vi "FMDLWaitKeithley6514ReadingBufferFull.vi"(0 "VISA resource name":refnum<visa-resource-name>, 1 "Timeout (10000 ms)":u32=10000, 2 "Buffer size previously set":i32, 3 "error in (no error)":errorcluster) -> (4 "Number of times the loop ran":i32, 5 "VISA resource name out":refnum<visa-resource-name>, 6 "Number of Readings in Buffer":i32, 7 "error out":errorcluster)   [LabVIEW 2018]
uses:
  <instrlib>/Keithley 6517/Keithley 6517.lvlib
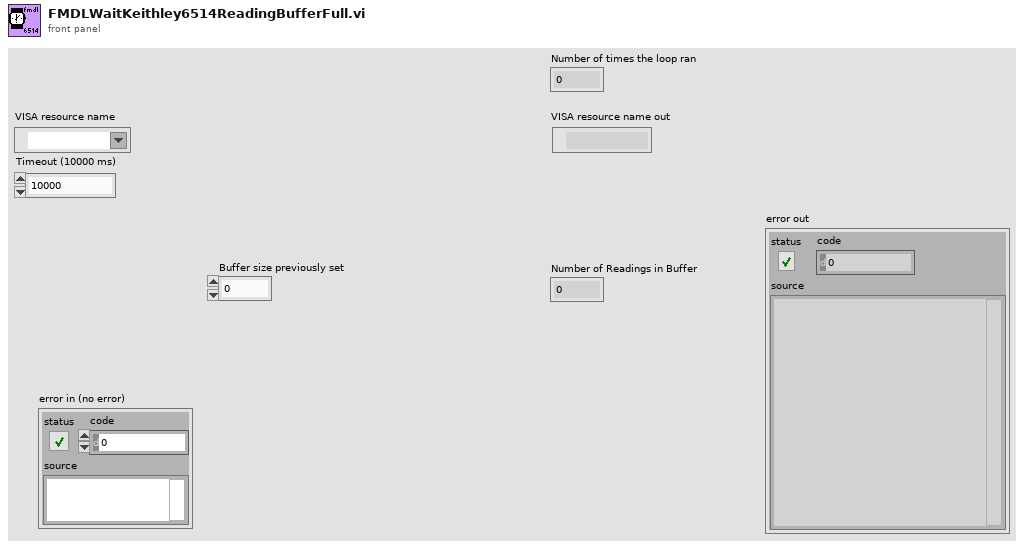
[diagram p1: front panel]
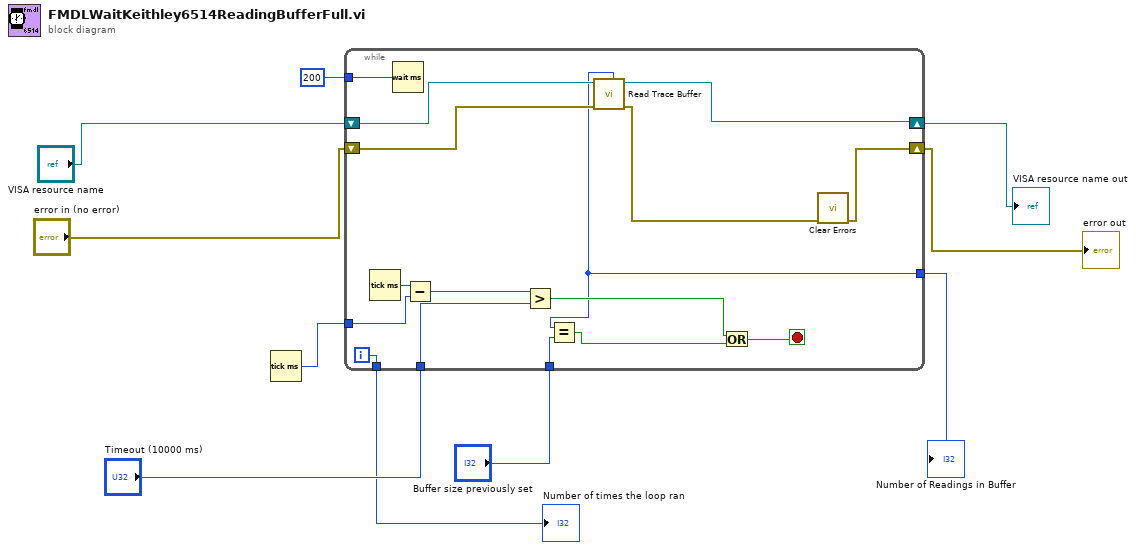
[diagram p0: block diagram]
diagram:
  n1 = Tick Count (ms)() -> (millisecond timer value=w8:u32)
  n2 = while {
    tunnel: 200 -> [w26]
    tunnel: w8 -> [w24]
    tunnel: "Timeout (10000 ms)" -> [w22]
    tunnel: "Buffer size previously set" -> [w21]
    shift-right: [w16] -> w4
    shift-left: "VISA resource name" -> [w18]
    shift-right: [w13] -> w6
    shift-left: "error in (no error)" -> [w17]
    tunnel: [w12] -> w3
    tunnel: [w11] -> w2
    i -> [w11]
    stop <- w20 stop-if-true
    n3 = Tick Count (ms)() -> (millisecond timer value=w25:u32)
    n4 = Wait (ms)(milliseconds to wait=w26) -> ()  [unwired: 1 out]
    n5 = Subtract(x=w25, y=w24) -> (x-y=w23:u32)
    n6 = Greater?(x=w23, y=w22) -> (0:w15:bool)
    n7 = call <instrlib>:"Read Trace Buffer.vi"("error in (no error)"=w17, "VISA resource name"=w18) -> ("error out"=w14:errorcluster, "VISA resource name out"=w16:refnum<visa-resource-name>, "Actual Trace Buffer Size"=w12:i32)  [unwired: 5 in, 2 out]
    n8 = Equal?(x=w12, y=w21) -> (x = y?=w19:bool)
    n9 = Or(x=w15, y=w19) -> (x .or. y?=w20:bool)
    n10 = call <vilib>:"Clear Errors.vi"("error in (no error)"=w14) -> ("error out"=w13:errorcluster)  [unwired: 5 in, 1 out]
  }
  "error out" <- w6
  "VISA resource name out" <- w4
  "Number of Readings in Buffer" <- w3
  "Number of times the loop ran" <- w2
